vi "FGV_DataPackerDebugMode.vi"(7 "?":T1, 11 "Boolean":bool=TRUE) -> (3 "Debug Mode":bool)   [LabVIEW 2018, in "feGEM DataPacker.lvlib"]
uses:
  feGEM DataPacker.lvlib
  Set_And_Get_Enum.ctl
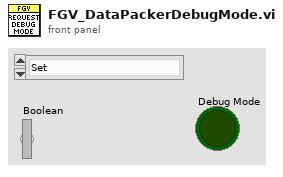
[diagram p1: front panel]
types:
  T1 = typedef "feGEM DataPacker.lvlib/Set_And_Get_Enum.ctl" = enum16{"Set", "Get"}
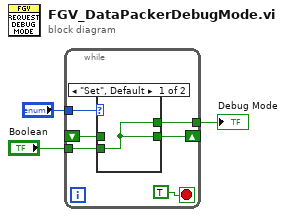
[diagram p0: block diagram]
diagram:
  n1 = while {
    tunnel: "Boolean" -> [w7]
    tunnel: [w8] -> w1
    shift-right: [w6] -> _
    shift-left: _ -> [w5]
    tunnel: "?" -> [w4]
    stop <- TRUE stop-if-true
    n2 = case shown="\"Set\", Default" w4 {
      tunnel: [w10 w11] -> w8
      tunnel: w7 -> [w10 _]
      tunnel: [w10 w11] -> w6
      tunnel: w5 -> [_ w11]
      frame "Set", Default {
      }
      frame "Get" {
      }
    }
  }
  "Debug Mode" <- w1
